vi "Convert Home Directory Tokens.vi"(11 "Home Directory Token":path) -> (3 "Home Directory":path)   [LabVIEW 2020, in "RxnRover.lvlib" / "User Preferences File.lvclass"]
doc: "Checks if a recognized home directory token was given and provides the home directory path using the built-in Get System Directory VI for the User Home directory. This VI will not create the directory if it does not exist and will not modify the given input token path if a valid token is not found."
uses:
  User Preferences File.lvclass
  <vilib>/Utility/sysdir.llb/System Directory Type.ctl
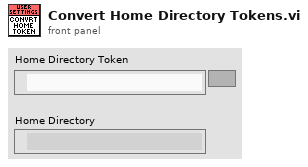
[diagram p1: front panel]
types:
  T1 = typedef "System Directory Type.ctl" = i32
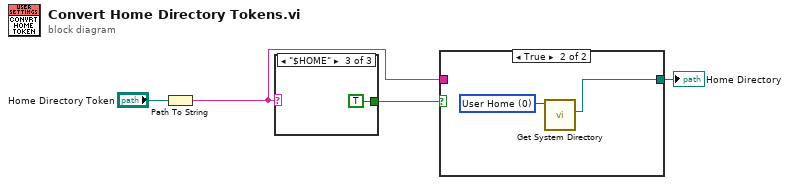
[diagram p0: block diagram]
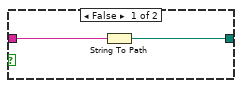
[diagram p2: hidden frame]
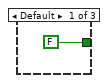
[diagram p3: hidden frame]
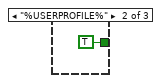
[diagram p4: hidden frame]
diagram:
  n1 = Path To String(path="Home Directory Token") -> (string=w2:string)
  n2 = case shown="\"$HOME\"" w2 {
    tunnel: [FALSE TRUE TRUE] -> w3
    frame Default {
    }
    frame "%USERPROFILE%" {
    }
    frame "$HOME" {
    }
  }
  n3 = case shown="True" w3 {
    tunnel: w2 -> [w9 _]
    tunnel: [w8 w10] -> w1
    frame False {
      n4 = String To Path(string=w9) -> (path=w8:path)
    }
    frame True {
      w11 = T1 0 items=["User Home"=0, "User Desktop"=1, "User Documents"=2, "User Application Data"=3, "User Preferences"=4, "User Temporary"=5, "Public Documents"=6, "Public Application Data"=7, "Public Preferences"=8, "Public Cache"=13, "System Core Libraries"=9, "System Installed Libraries"=10, "Application Files"=11, "Boot Volume Root"=12] ("system directory type")
      n5 = call <vilib>:"Get System Directory.vi"("system directory type"=w11) -> ("system directory"=w10:path)  [unwired: 10 in]
    }
  }
  "Home Directory" <- w1
